vi "导出基准数据.vi"(8 "error in":errorcluster, 9 "OUT":i32=4, 11 "IN":i32=128) -> (0 "error out":errorcluster)   [LabVIEW 2015]
uses:
  server/Global/SeverGlobal.vi
  <vilib>/Utility/NIReport.llb/NI_report.lvclass
  <vilib>/Utility/NIReport.llb/Excel/NI_Excel.lvclass
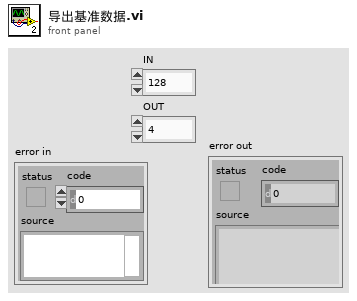
[diagram p1: front panel]
types:
  T1 = enum16{"Standard Report", "HTML", "Word", "Excel"}
  T2 = enum16{"maximized", "minimized", "normal", "no change"}
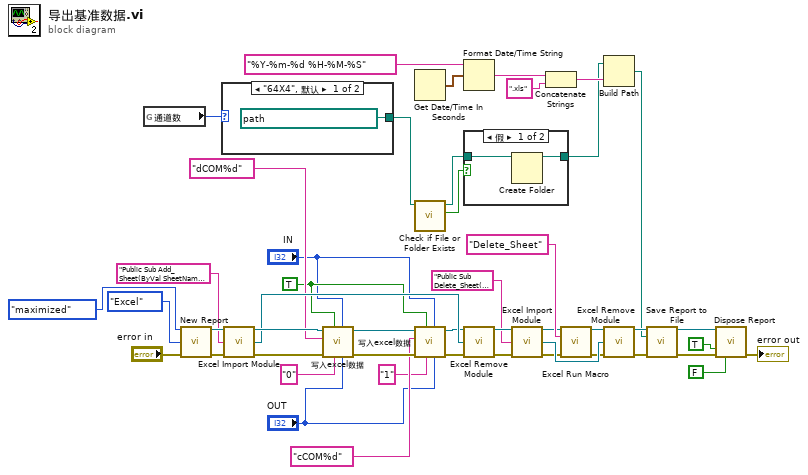
[diagram p0: block diagram]
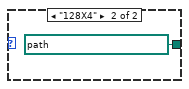
[diagram p2: hidden frame]
diagram:
  w5 = TRUE ("ref")
  n1 = global read "SeverGlobal.vi" "通道数"() -> (w2:enum16{"64X4", "128X4"})
  n2 = call <vilib>:"New Report.vi"("window state (normal)"=T2."maximized", "report type"=T1."Excel", "error in (no error)"="error in") -> ("report out"=w46:refnum<class "NI_report.lvclass">, "error out"=w47:errorcluster)  [unwired: 11 in]
  n3 = case shown="\"64X4\", 默认" w2 {
    tunnel: [path "D:/64X4数据/基准数据" ("base path") path "D:/128X4数据/基准数据" ("base path")] -> w1
    frame "64X4", Default {
    }
    frame "128X4" {
    }
  }
  n4 = call <vilib>:"Excel Import Module.vi"("report in"=w46, "module code (\"\")"="Public Sub Add_Sheet(ByVal SheetName As String)\n    Dim shcount As Integer\n    shcount = Sheets.Count\n    Sheets.Add after:=Sheets(shcount)\n    shcount = shcount + 1\n    Sheets(shcount).Name = SheetName\nEnd Sub" ("module code (\"\")"), "error in (no error)"=w47) -> ("report out"=w41:refnum<class "NI_report.lvclass">, "module reference"=w17:refnum<k7>, "error out"=w40:errorcluster)  [unwired: 10 in]
  n5 = call "写入excel数据.vi"("OUT"="OUT", "IN"="IN", "testType"="0", "ref"=w5, "error in (no error)"=w40, "style"="dCOM%d", "NI_report in"=w41) -> ("error out"=w14:errorcluster, "NI_report out"=w15:refnum<class "NI_report.lvclass">)  [unwired: 3 in]
  n6 = Get Date/Time In Seconds() -> (seconds since 1Jan1904=w19:timestamp)
  n7 = call <vilib>:"Check if File or Folder Exists.vi"("path"=w1) -> ("file or folder exists?"=w10:bool, "dup path"=w9:path)  [unwired: 8 in, 1 out]
  n8 = call "写入excel数据.vi"("OUT"="OUT", "IN"="IN", "testType"="1", "ref"=w5, "error in (no error)"=w14, "style"="cCOM%d", "NI_report in"=w15) -> ("error out"=w13:errorcluster, "NI_report out"=w12:refnum<class "NI_report.lvclass">)  [unwired: 3 in]
  n9 = Format Date/Time String(time format string (%c)="%Y-%m-%d %H-%M-%S", seconds (now)=w19) -> (date/time string=w22:string)  [unwired: 1 in]
  n10 = case shown="假" w10 {
    tunnel: w9 -> [w51 w52]
    tunnel: [w50 w52] -> w8
    frame False {
      n11 = Create Folder(path (use dialog)=w51) -> (created path=w50:path)  [unwired: 2 in, 2 out]
    }
    frame True {
    }
  }
  n12 = call <vilib>:"Excel Remove Module.vi"("report in"=w12, "module reference"=w17, "error in (no error)"=w13) -> ("report out"=w31:refnum<class "NI_report.lvclass">, "error out"=w32:errorcluster)  [unwired: 11 in]
  n13 = call <vilib>:"Excel Import Module.vi"("report in"=w31, "module code (\"\")"="Public Sub Delete_Sheet()\n    Application.DisplayAlerts = False\nSheets(\"Sheet1\").Delete\n    Sheets(\"Sheet2\").Delete\n    Sheets(\"Sheet3\").Delete\n    Application.DisplayAlerts = True\nEnd Sub" ("module code (\"\")"), "error in (no error)"=w32) -> ("report out"=w25:refnum<class "NI_report.lvclass">, "module reference"=w30:refnum<k7>, "error out"=w26:errorcluster)  [unwired: 10 in]
  n14 = Concatenate Strings(w22, ".xls") -> (w23:string)
  n15 = call <vilib>:"Excel Run Macro.vi"("report in"=w25, "macro name"="Delete_Sheet", "error in (no error)"=w26) -> ("report out"=w28:refnum<class "NI_report.lvclass">, "error out"=w29:errorcluster)  [unwired: 10 in, 1 out]
  n16 = Build Path(base path=w8, name or relative path=w23) -> (appended path=w18:path)
  n17 = call <vilib>:"Excel Remove Module.vi"("report in"=w28, "module reference"=w30, "error in (no error)"=w29) -> ("report out"=w33:refnum<class "NI_report.lvclass">, "error out"=w34:errorcluster)  [unwired: 11 in]
  n18 = call-dynamic "Save Report to File.vi"("report in"=w33, "report file path"=w18, "error in (no error)"=w34) -> ("report out"=w35:refnum<class "NI_report.lvclass">, "error out"=w36:errorcluster)  [unwired: 11 in]
  n19 = call-dynamic "Dispose Report.vi"("report in"=w35, "save changes? (F)"=TRUE, "error in (no error)"=w36, "close report? (T)"=FALSE) -> ("error out"=→"error out":errorcluster)  [unwired: 11 in]
